vi "display lines.vi"(8 "error in (no error)":errorcluster, 11 "Arduino Uno in":refnum<class "Arduino Uno.lvclass">) -> (0 "error out":errorcluster, 1 "Values":i32[](array[numeric]), 2 "Lines":string[](array[string]), 3 "Arduino Uno out":refnum<class "Arduino Uno.lvclass">)   [LabVIEW 2025, in "USB IO.lvlib" / "Arduino Uno.lvclass"]
uses:
  Arduino Uno.lvclass
  Arduino Uno.lvclass/Arduino Uno.ctl
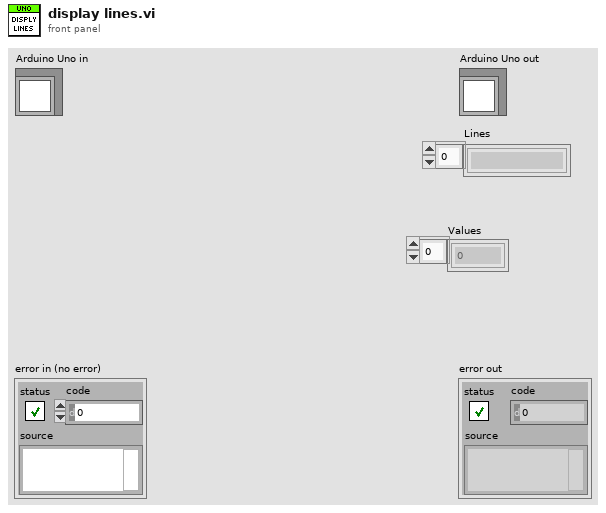
[diagram p1: front panel]
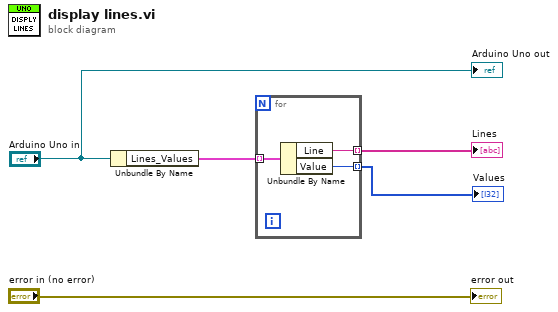
[diagram p0: block diagram]
diagram:
  n1 = Unbundle By Name("Arduino Uno in") -> ("Lines_Values"=w5:cluster{"Line":string, "Value":i32}[])
  n2 = for {
    tunnel: w5 -> [w8] mode=indexing
    tunnel: [w7] -> w3 mode=indexing
    tunnel: [w6] -> w1 mode=indexing
    n3 = Unbundle By Name(w8) -> ("Line"=w7:string, "Value"=w6:i32)
  }
  "Lines" <- w3
  "Values" <- w1
  "error out" <- "error in (no error)"
  "Arduino Uno out" <- "Arduino Uno in"
